vi "Range Array Constants.vi"(7 "Triggered Mode":T1, 8 "error in (no error)":errorcluster, 10 "Triggered?":bool, 11 "3300 in":refnum<class "3300.lvclass">) -> (0 "error out":errorcluster, 2 "Range Array":dbl[](array[numeric]), 3 "3300 out":refnum<class "3300.lvclass">)   [LabVIEW 2019, in "3300.lvlib" / "3300.lvclass"]
uses:
  Library/3300.lvclass
  C:/Users/Public/Documents/Development/builds/Instruments/Electronic Load.lvlibp/Library/Electronic Load.lvclass
  builds/Instruments/Electronic Load.lvlibp/Custom Controls/E-Load Mode.ctl
  builds/Instruments/Electronic Load.lvlibp/Accessors/Trigger/Read Pulse Mode.vi
  Accessors/Read Active Module.vi
  builds/Instruments/Electronic Load.lvlibp/Library/Electronic Load.lvclass
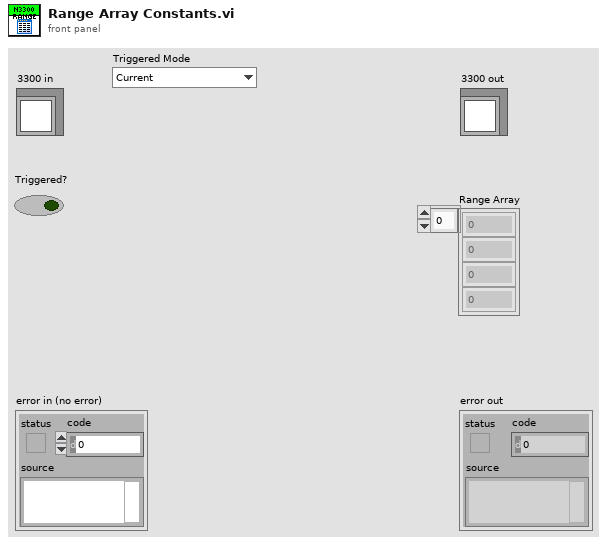
[diagram p1: front panel]
types:
  T1 = typedef "Electronic Load.lvlibp/Electronic Load.lvclass/E-Load Mode.ctl" = enum16{"Current", "Resistance", "Voltage"}
  T2 = typedef "3300.lvlib/3300.lvclass/Modules.ctl" = enum16{"N3302A", "N3303A", "N3304A", "N3305A", "N3306A", "N3307A"}
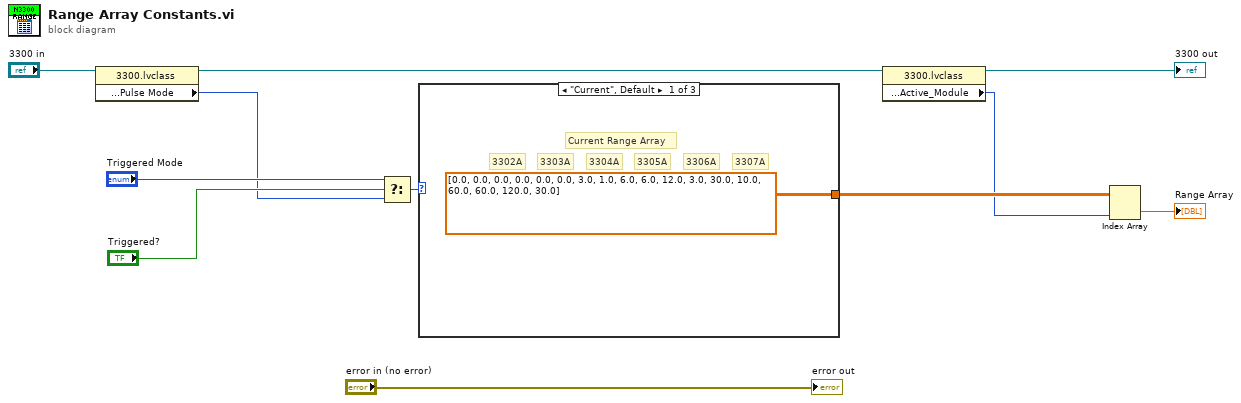
[diagram p0: block diagram]
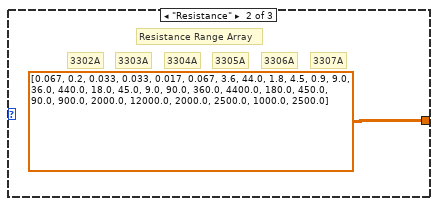
[diagram p2: hidden frame]
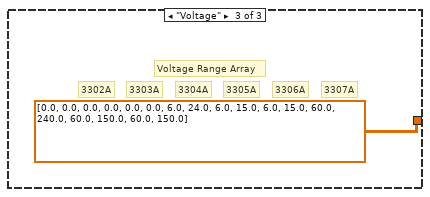
[diagram p3: hidden frame]
diagram:
  n1 = property class="3300.lvclass"(reference="3300 in") -> (reference out=w6:refnum<class "3300.lvclass">, "Accessors:Settings:Pulse:Pulse Mode"=w1:T1)  [unwired: 1 in, 1 out]
  n2 = Select(t="Triggered Mode", s="Triggered?", f=w1) -> (s? t:f=w5:T1)
  n3 = case shown="\"Current\", Default" w5 {
    tunnel: [dbl[][] [[0.0, 0.0, 0.0, 0.0, 0.0, 0.0], [3.0, 1.0, 6.0, 6.0, 12.0, 3.0], [30.0, 10.0, 60.0, 60.0, 120.0, 30.0]] dbl[][] [[0.067, 0.2, 0.033, 0.033, 0.017, 0.067], [3.6, 44.0, 1.8, 4.5, 0.9, 9.0], [36.0, 440.0, 18.0, 45.0, 9.0, 90.0], [360.0, 4400.0, 180.0, 450.0, 90.0, 900.0], [2000.0, 12000.0, 2000.0, 2500.0, 1000.0, 2500.0]] dbl[][] [[0.0, 0.0, 0.0, 0.0, 0.0, 0.0], [6.0, 24.0, 6.0, 15.0, 6.0, 15.0], [60.0, 240.0, 60.0, 150.0, 60.0, 150.0]]] -> w9
    frame "Current", Default {
      # "3307A"
      # "3306A"
      # "3305A"
      # "3304A"
      # "3303A"
      # "3302A"
      # "Current Range Array"
    }
    frame "Resistance" {
      # "Resistance Range Array"
      # "3307A"
      # "3306A"
      # "3305A"
      # "3304A"
      # "3303A"
      # "3302A"
    }
    frame "Voltage" {
      # "3307A"
      # "3306A"
      # "3305A"
      # "3304A"
      # "3303A"
      # "3302A"
      # "Voltage Range Array"
    }
  }
  n4 = property class="3300.lvclass"(reference=w6) -> (reference out=→"3300 out":refnum<class "3300.lvclass">, "Private:Accessors:Active_Module"=w2:T2)  [unwired: 1 in, 1 out]
  n5 = Index Array(array=w9, index (col)=w2) -> (element=→"Range Array":dbl[])  [unwired: 1 in]
  "error out" <- "error in (no error)"
